vi "Send MSG to printer.vi"(8 "error in (no error)":errorcluster, 11 "Domino Laser module Class in":refnum<class "Domino Laser module Class.lvclass">) -> (0 "error out":errorcluster, 2 "Recived message":string, 3 "Domino Laser module Class out":refnum<class "Domino Laser module Class.lvclass">)   [LabVIEW 2024, in "Domino LM.lvlib" / "Domino Laser module Class.lvclass"]
uses:
  CTRLS/Domino Laser module Class.lvclass
  CTRLS/Domino Laser module Class.lvclass/Domino Laser module Class.ctl
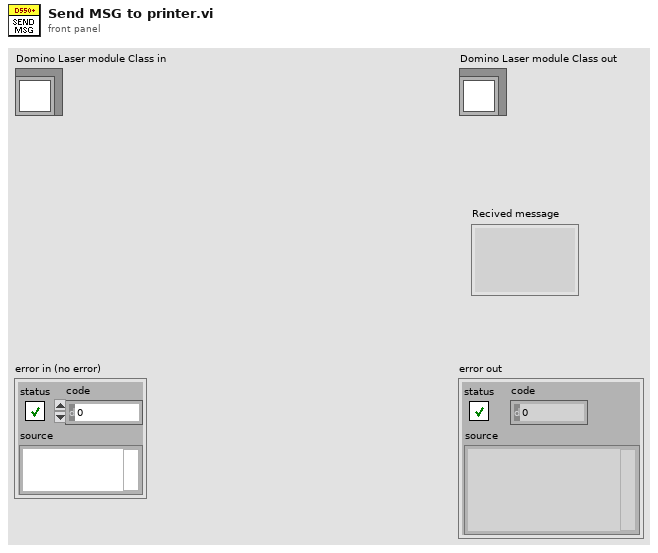
[diagram p1: front panel]
types:
  T1 = enum16{"Standard", "Buffered", "CRLF", "Immediate"}
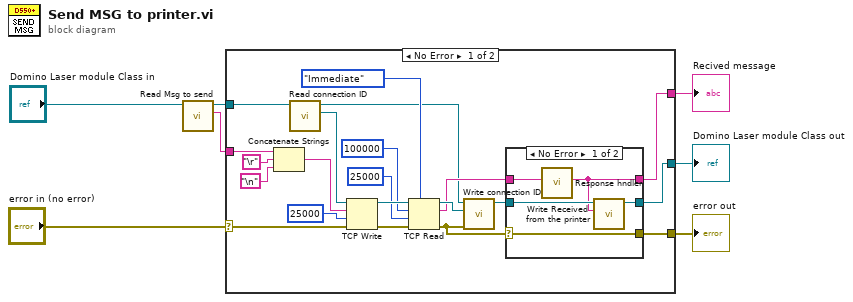
[diagram p0: block diagram]
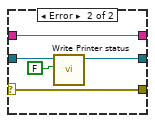
[diagram p2: hidden frame]
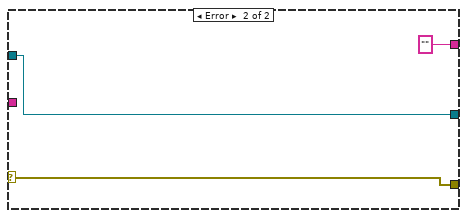
[diagram p3: hidden frame]
diagram:
  n1 = call "Read Msg to send.vi"("Domino Laser module Class in"="Domino Laser module Class in") -> ("Msg to send"=w3:string, "Domino Laser module Class out"=w2:refnum<class "Domino Laser module Class.lvclass">)  [unwired: 8 in, 1 out]
  n2 = case shown="No Error" "error in (no error)" {
    selector: "error in (no error)" -> [w12 w41]
    tunnel: [w11 w41] -> w6
    tunnel: [w16 w40] -> w5
    tunnel: w2 -> [w28 w40]
    tunnel: w3 -> [w27 _]
    tunnel: [w10 "" ("data out")] -> w1
    frame No Error {
      n3 = Concatenate Strings(w27, "\r", "\n") -> (w23:string)
      n4 = call "Read connection ID.vi"("Domino Laser module Class in"=w28) -> ("connection ID"=w24:refnum<k5>, "Domino Laser module Class out"=w14:refnum<class "Domino Laser module Class.lvclass">)  [unwired: 8 in, 1 out]
      n5 = TCP Write(connection ID=w24, data in=w23, error in (no error)=w12, 9:25000 ("timeout ms (25000)")) -> (connection ID out=w20:refnum<k5>, error out=w21:errorcluster)  [unwired: 1 out]
      n6 = TCP Read(connection ID=w20, bytes to read=100000 ("timeout ms (25000)"), error in (no error)=w21, 7:T1."Immediate" ("mode (standard)"), 9:25000 ("timeout ms (25000)")) -> (connection ID out=w18:refnum<k5>, data out=w15:string, error out=w13:errorcluster)
      n7 = call "Write connection ID.vi"("error in (no error)"=w13, "connection ID"=w18, "Domino Laser module Class in"=w14) -> ("Domino Laser module Class out"=w17:refnum<class "Domino Laser module Class.lvclass">)  [unwired: 7 in, 1 out]
      n8 = case shown="No Error" w13 {
        selector: w13 -> [w30 w35]
        tunnel: w17 -> [w32 w37]
        tunnel: [w31 w36] -> w16
        tunnel: w15 -> [w33 w34]
        tunnel: [w30 w35] -> w11
        tunnel: [w29 w34] -> w10
        frame No Error {
          n9 = call "Response hndler.vi"("Recived MSG"=w33) -> ("printer response"=w29:string)  [unwired: 8 in, 2 out]
          n10 = call "Write Received from the printer.vi"("Received from the printer"=w29, "Domino Laser module Class in"=w32) -> ("Domino Laser module Class out"=w31:refnum<class "Domino Laser module Class.lvclass">)  [unwired: 8 in, 1 out]
        }
        frame Error {
          n11 = call "Write Printer status.vi"("Printer status"=FALSE, "Domino Laser module Class in"=w37) -> ("Domino Laser module Class out"=w36:refnum<class "Domino Laser module Class.lvclass">)  [unwired: 8 in, 1 out]
        }
      }
    }
    frame Error {
    }
  }
  "error out" <- w6
  "Domino Laser module Class out" <- w5
  "Recived message" <- w1
